vi "TCP_echo.vi"() -> ()   [LabVIEW 2014]
uses:
  <vilib>/Utility/error.llb/DialogType.ctl
panel:
  out "Client connected":bool
  in  "DataSocket Target":string="dstp://localhost/currentsources"
  out "volts":dbl[](array[numeric])
  in  "stop when client stops":bool
  out "response":string
  out "request":string
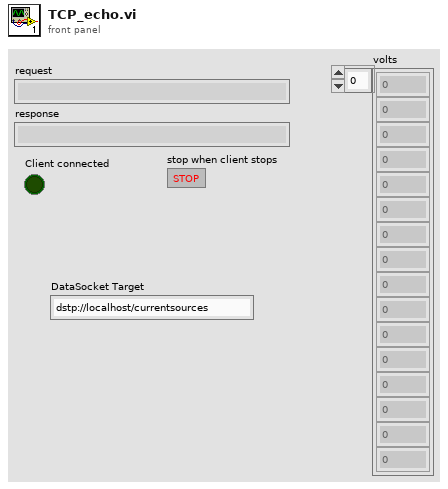
[diagram p1: front panel]
types:
  T1 = enum16{"Read", "Write", "ReadWrite", "BufferedRead", "BufferedReadWrite"}
  T2 = enum16{"Standard", "Buffered", "CRLF", "Immediate"}
  T3 = typedef "DialogType.ctl" = u16
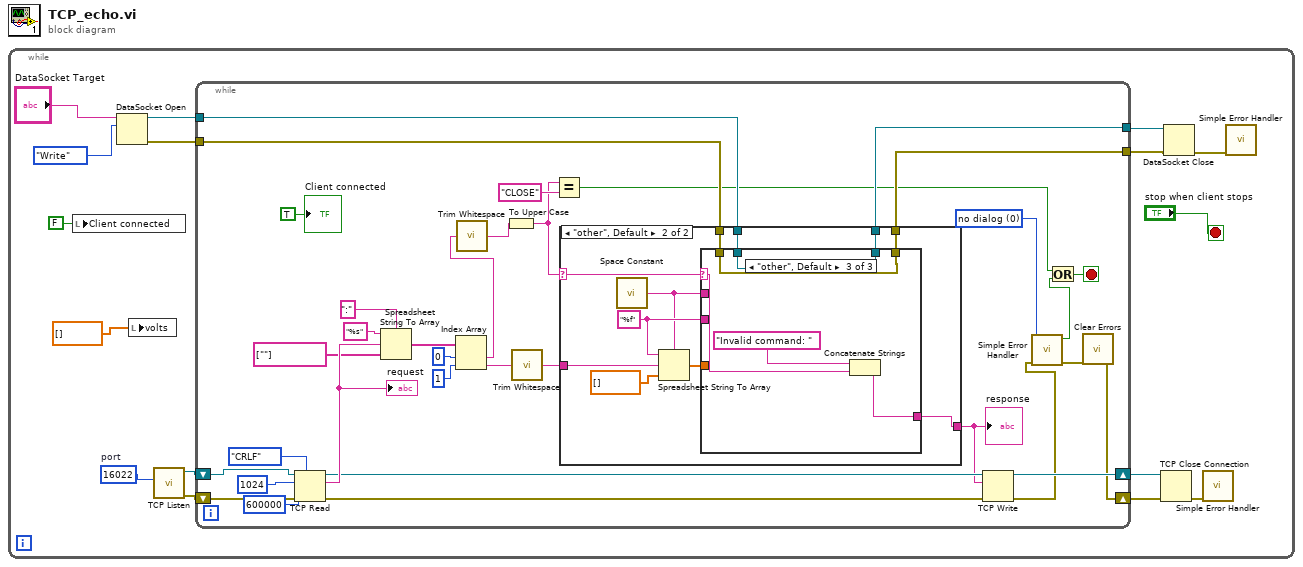
[diagram p0: block diagram]
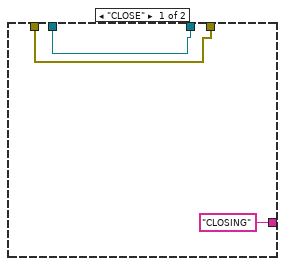
[diagram p2: hidden frame]
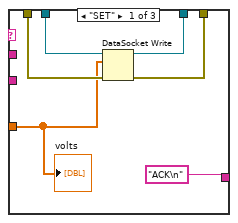
[diagram p3: hidden frame]
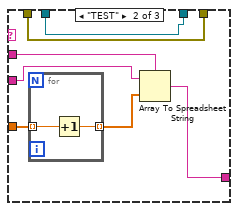
[diagram p4: hidden frame]
diagram:
  n1 = while {
    stop <- "stop when client stops" stop-if-true
    w11 = u16 16022  # port
    n2 = local write "Client connected"(FALSE ("Client connected")) -> ()
    n3 = DataSocket Open(10:T1."Write" ("mode"), 11:"DataSocket Target") -> (0:w5:errorcluster, 3:w4:refnum<k13>)  [unwired: 2 in]
    n4 = local write "volts"(dbl[] []) -> ()
    n5 = call <vilib>:"TCP Listen.vi"("port"=w11) -> ("error out"=w15:errorcluster, "connection ID"=w16:refnum<k5>)  [unwired: 6 in, 3 out]
    n6 = while {
      shift-right: [w38] -> w14
      shift-left: w16 -> [w50]
      shift-right: [w20] -> w13
      shift-left: w15 -> [w49]
      tunnel: w4 -> [w29]
      tunnel: w5 -> [w28]
      tunnel: [w27] -> w2
      tunnel: [w26] -> w1
      stop <- w25 stop-if-true
      w19 = T3 0 items=["no dialog", "OK message", "continue or stop message", "OK message + warnings", "continue/stop + warnings"] ("type of dialog (OK msg:1)")
      n7 = TCP Read(connection ID=w50, bytes to read=1024, error in (no error)=w49, 7:T2."CRLF" ("mode (standard)"), 9:600000 ("timeout ms (25000)")) -> (connection ID out=w36:refnum<k5>, data out=w46:string, error out=w37:errorcluster)
      "request" <- w46
      n8 = Spreadsheet String To Array(delimiter (Tab)=":", format string="%s", spreadsheet string=w46, array type (2D Dbl)=string[] [""]) -> (array=w44:string[])
      n9 = Index Array(array=w44, index #1=0 ("index"), index #2=1 ("index")) -> (element #1=w41:string, element #2=w31:string)
      n10 = call <vilib>:"Trim Whitespace.vi"("string"=w41) -> ("trimmed string"=w33:string)  [unwired: 1 in]
      n11 = To Upper Case(1:w33) -> (0:w32:string)
      n12 = call <vilib>:"Trim Whitespace.vi"("string"=w31) -> ("trimmed string"=w30:string)  [unwired: 1 in]
      n13 = Equal?(x=w32, y="CLOSE") -> (x = y?=w24:bool)
      n14 = case shown="\"other\", Default" w32 {
        selector: w32 -> [_ w59]
        tunnel: w30 -> [_ w60]
        tunnel: ["CLOSING" w58] -> w35
        tunnel: w29 -> [w52 w57]
        tunnel: w28 -> [w51 w56]
        tunnel: [w52 w55] -> w27
        tunnel: [w51 w54] -> w26
        frame "CLOSE" {
        }
        frame "other", Default {
          w64 = "%f" ("format string")
          n15 = call <vilib>:"Space Constant.vi"() -> ("String"=w63:string)
          n16 = Spreadsheet String To Array(delimiter (Tab)=w63, format string=w64, spreadsheet string=w60, array type (2D Dbl)=dbl[] []) -> (array=w62:dbl[])
          n17 = case shown="\"other\", Default" w59 {
            selector: w59 -> [_ _ w83]
            tunnel: w64 -> [_ w77 _]
            tunnel: w63 -> [_ w76 _]
            tunnel: w62 -> [w65 w74 _]
            tunnel: ["ACK\n" ("spreadsheet string") w73 w82] -> w58
            tunnel: w57 -> [w69 w72 w81]
            tunnel: w56 -> [w68 w71 w80]
            tunnel: [w67 w72 w81] -> w55
            tunnel: [w66 w71 w80] -> w54
            frame "SET" {
              n18 = DataSocket Write(8:w68, 10:w65, 11:w69) -> (0:w66:errorcluster, 3:w67:refnum<k13>)  [unwired: 1 in, 1 out]
              "volts" <- w65
            }
            frame "TEST" {
              n19 = for {
                tunnel: w74 -> [w79] mode=indexing
                tunnel: [w78] -> w75 mode=indexing
                n20 = Increment(x=w79) -> (x+1=w78:dbl)
              }
              n21 = Array To Spreadsheet String(delimiter (Tab)=w76, array=w75, 3:w77) -> (spreadsheet string=w73:string)
            }
            frame "other", Default {
              n22 = Concatenate Strings("Invalid command: ", w83) -> (w82:string)
            }
          }
        }
      }
      "response" <- w35
      n23 = TCP Write(connection ID=w36, data in=w35, error in (no error)=w37) -> (connection ID out=w38:refnum<k5>, error out=w21:errorcluster)  [unwired: 2 out]
      n24 = call <vilib>:"Simple Error Handler.vi"("type of dialog (OK msg:1)"=w19, "error in (no error)"=w21) -> ("error?"=w23:bool, "error out"=w22:errorcluster)  [unwired: 3 in, 3 out]
      n25 = Or(x=w24, y=w23) -> (x .or. y?=w25:bool)
      n26 = call <vilib>:"Clear Errors.vi"("error in (no error)"=w22) -> ("error out"=w20:errorcluster)  [unwired: 5 in, 1 out]
      "Client connected" <- TRUE ("Client connected")
    }
    n27 = TCP Close Connection(connection ID=w14, error in (no error)=w13) -> (error out=w12:errorcluster)  [unwired: 1 in, 1 out]
    n28 = DataSocket Close(8:w1, 11:w2) -> (0:w3:errorcluster)  [unwired: 1 in, 1 out]
    n29 = call <vilib>:"Simple Error Handler.vi"("error in (no error)"=w12) -> ()  [unwired: 4 in, 5 out]
    n30 = call <vilib>:"Simple Error Handler.vi"("error in (no error)"=w3) -> ()  [unwired: 4 in, 5 out]
  }
